vi "Math Find Fano Factor.vi"(8 "Error In":errorcluster, 10 "Fitted Values":dbl[](array[numeric]), 11 "Y Array":dbl[](array[numeric])) -> (0 "Error Out":errorcluster, 3 "Fano Factor":dbl)   [LabVIEW 2021, in "Math.lvlib"]
uses:
  Math.lvlib
  Math Fano Factor Zero Finder Data.ctl
  Fano Factor Zero Finder f(x) 1D.vi
  <vilib>/gmath/zero.llb/Newton Raphson Zero Finder (VI).vi
  <vilib>/gmath/NI_Gmath.lvlib
  Error/Error.lvlib
panel:
  out "Minimum":dbl
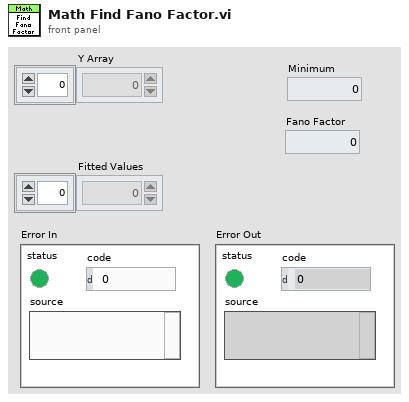
[diagram p1: front panel]
types:
  T1 = typedef "Math.lvlib/Math Fano Factor Zero Finder Data.ctl" = cluster{"Data":dbl[], "Fit":dbl[]}
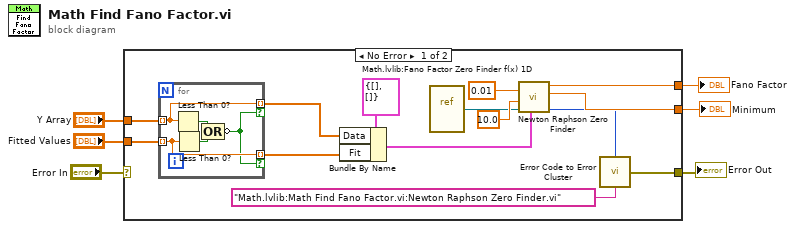
[diagram p0: block diagram]
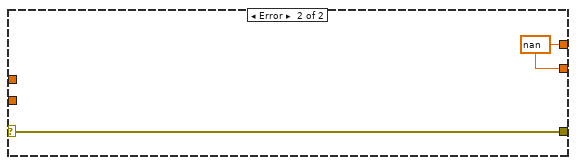
[diagram p2: hidden frame]
diagram:
  n1 = case shown="No Error" "Error In" {
    selector: "Error In" -> [_ w27]
    tunnel: "Y Array" -> [w20 _]
    tunnel: "Fitted Values" -> [w19 _]
    tunnel: [w13 w26] -> w4
    tunnel: [w8 w27] -> w2
    tunnel: [w12 w26] -> w1
    frame No Error {
      n2 = for {
        tunnel: w20 -> [w23] mode=indexing
        tunnel: w19 -> [w22] mode=indexing
        tunnel: [w23] -> w18 mode=indexing if=w21
        tunnel: [w22] -> w17 mode=indexing if=w21
        n3 = Less Than 0?(x=w23) -> (x < 0?=w25:bool)
        n4 = Less Than 0?(x=w22) -> (x < 0?=w24:bool)
        n5 = Compound Arithmetic op=OR(w25, w24) -> (invert w21:bool)
      }
      n6 = Bundle By Name(cluster=T1 {"Data"=[], "Fit"=[]} ("output cluster"), "Data"=w18, "Fit"=w17) -> (w10:T1)
      n7 = vi-ref "Math.lvlib:Fano Factor Zero Finder f(x) 1D.vi"() -> (w11:refnum<vi>)
      n8 = call-poly <vilib>:"Newton Raphson Zero Finder.vi"("data"=w10, "f(x)"=w11, "end"=10.0, "start"=0.01) -> ("error"=w9:i32, "f(zero)"=w12:dbl, "zero"=w13:dbl)  [unwired: 4 in, 1 out]
      n9 = call "Error Code to Error Cluster.vi"("Error Code"=w9, "Error Source"="Math.lvlib:Math Find Fano Factor.vi:Newton Raphson Zero Finder.vi") -> ("Error Out"=w8:errorcluster)  [unwired: 13 in]
    }
    frame Error {
      w26 = nan ("zero")
    }
  }
  "Fano Factor" <- w4
  "Error Out" <- w2
  "Minimum" <- w1
